vi "LV SCISDK Read Spectrum Data.vi"(0 "Path 2":string, 2 "handle 2":u64, 3 "error in (no error) 2":errorcluster) -> (7 "error out 2":errorcluster, 8 "buffer out":T1, 9 "handle out 2":u64, 10 "function return 2":i32)   [LabVIEW 2021, in "SciSDK_Labview.lvlib"]
doc: "SCISDKLABVIEW_DLL_API int LV_SCISDK_ReadSpectrum(char* Path, TD_SPECTRUM* buffer, void* handle);"
uses:
  SciSDK_Labview.lvlib
  SciSDK_VC++/x64/Debug/SciSDK_Labview.dll
panel:
  in  "buffer":T1={"magic"=0, "timecode"=0, "inttime"=0, "buffer_size"=0, "total_bins"=0, "valid_bins"=0, "data"=[10, 100]}
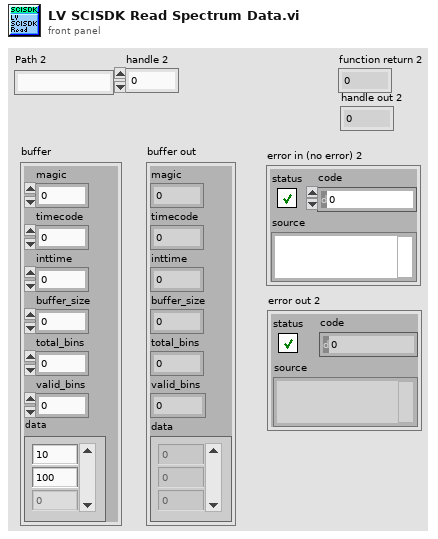
[diagram p1: front panel]
types:
  T1 = cluster{"magic":u32, "timecode":u32, "inttime":u32, "buffer_size":u32, "total_bins":u32, "valid_bins":u32, "data":i32[]}
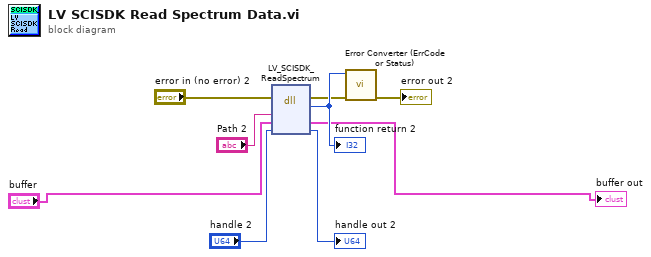
[diagram p0: block diagram]
diagram:
  n1 = dll-call lib="C:/git/scisdk/SciSDK_VC++/x64/Debug/SciSDK_Labview.dll" fn="LV_SCISDK_ReadSpectrum"(error in="error in (no error) 2", "Path"="Path 2", "buffer"="buffer", "handle"="handle 2") -> (error out=w4:errorcluster, "return type"=w9:i32, "buffer"=→"buffer out":T1, "handle"=→"handle out 2":u64)  [unwired: 3 in, 1 out]
  "function return 2" <- w9
  n2 = call <userlib>:"Error Converter (ErrCode or Status).vi"("error in (no error)"=w4, "error code"=w9) -> ("error out"=→"error out 2":errorcluster)  [unwired: 9 in]
